vi "Global_Vision Server Data.vi"() -> ()   [LabVIEW 2017, in "VisionSystem.lvlib"]
uses:
  VisionSystem.lvlib
  TypeDefs/Cluster_Camera Settings.ctl
  <vilib>/Rock Robotics/WPI/Camera/WPI_CameraImageSize.ctl
  <vilib>/Rock Robotics/WPI/Camera/WPI_CameraFrameRate.ctl
  <vilib>/Rock Robotics/WPI/Camera/WPI_CameraWhite Balance Values.ctl
  <vilib>/Rock Robotics/WPI/Camera/WPI_CameraExposure Values.ctl
panel:
  in  "Compression":i32
  in  "Vision Server_Camera Settings":T1={"Image Size"=enum."160x120", "Frame Rate (fps)"=0, "White Balance"=enum."Auto", "Exposure"=enum."Auto", "Exposure (%)"=0.0, "Brightness"=0, "Sharpness"=0, "Saturation"=0} {"Saturation" min=0 max=100 step=1; "Sharpness" min=0 max=100 step=1; "Brightness" min=0 max=100 step=1; "Exposure (%)" min=0.0 max=100.0 step=1.0}
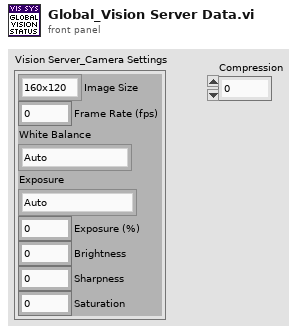
[diagram p1: front panel]
types:
  T1 = typedef "Cluster_Camera Settings.ctl" = cluster{"Image Size":T2, "Frame Rate (fps)":T3, "White Balance":T4, "Exposure":T5, "Exposure (%)":dbl, "Brightness":i32, "Sharpness":i32, "Saturation":i32}
  T2 = typedef "WPI_CameraImageSize.ctl" = enum16{"640x480", "320x240", "160x120", "Custom"}
  T3 = typedef "WPI_CameraFrameRate.ctl" = u32
  T4 = typedef "WPI_CameraWhite Balance Values.ctl" = enum16{"Auto", "Fixed indoor", "Fixed outdoor 1", "Fixed outdoor 2", "Fixed fluorescent 1", "Fixed fluorescent 2", "Hold current", "Custom"}
  T5 = typedef "WPI_CameraExposure Values.ctl" = enum16{"Auto", "Flicker-free 50 Hz", "Flicker-free 60 Hz", "Hold current", "Custom"}
diagram:
